vi "Local qubit state.vi"(11 "Circuit cluster":T1) -> (3 "Local qubit state":cdb[](array[numeric]))   [LabVIEW 2016]
doc: "*Local state vector is only valid for non-entangled qubits"
uses:
  TypeDefs/Circuit Cluster.ctl
  Classes/GateAbst/GateAbst.lvclass
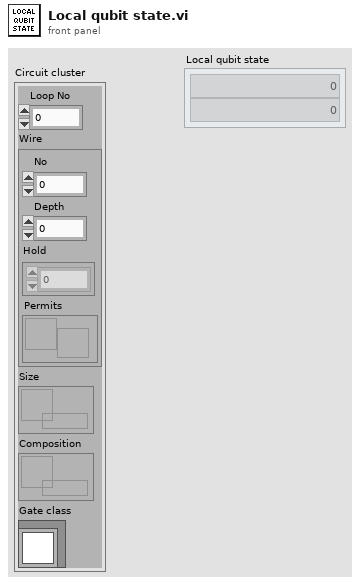
[diagram p1: front panel]
types:
  T1 = typedef "Circuit Cluster.ctl" = cluster{"Loop No":i32, "Wire":cluster{"No":i32, "Depth":i32, "Hold":i32[][], "Permits":refnum<notifier>}, "Size":refnum<queue>, "Composition":refnum<queue>, "Gate class":refnum<class "GateAbst.lvclass">}
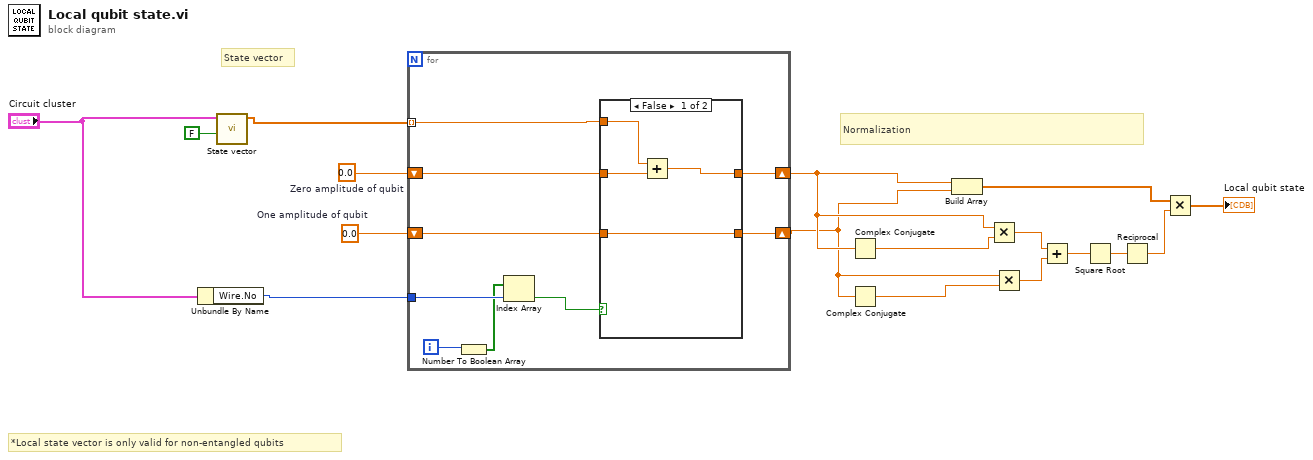
[diagram p0: block diagram]
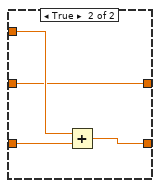
[diagram p2: hidden frame]
diagram:
  w14 = 0.0  # One amplitude of qubit
  w15 = 0.0  # Zero amplitude of qubit
  # "*Local state vector is only valid for non-entangled qubits"
  # "Normalization"
  # "State vector"
  n1 = Unbundle By Name("Circuit cluster") -> ("Wire.No"=w17:i32)
  n2 = call "State vector.vi"("Final state? (T)"=FALSE ("Final state?"), "Circuit cluster"="Circuit cluster") -> ("State vector"=w3:cdb[])  [unwired: 9 in]
  n3 = for {
    tunnel: w17 -> [w25]
    tunnel: w3 -> [w22] mode=indexing
    shift-right: [w18] -> w10
    shift-left: w14 -> [w19]
    shift-right: [w20] -> w11
    shift-left: w15 -> [w21]
    i -> [w26]
    n4 = Number To Boolean Array(number=w26) -> (Boolean array=w24:bool[])
    n5 = Index Array "Index Array"(array=w24, index=w25) -> (element=w23:bool)
    n6 = case shown="False" w23 {
      tunnel: w22 -> [w30 w34]
      tunnel: w21 -> [w29 w31]
      tunnel: [w28 w31] -> w20
      tunnel: w19 -> [w27 w33]
      tunnel: [w27 w32] -> w18
      frame False {
        n7 = Add(x=w30, y=w29) -> (x+y=w28:cdb)
      }
      frame True {
        n8 = Add(x=w34, y=w33) -> (x+y=w32:cdb)
      }
    }
  }
  n9 = Complex Conjugate(1:w11) -> (0:w16:cdb)
  n10 = Complex Conjugate(1:w10) -> (0:w13:cdb)
  n11 = Build Array "Build Array"(w11, w10) -> (w7:cdb[])
  n12 = Multiply(x=w11, y=w16) -> (x*y=w5:cdb)
  n13 = Multiply(x=w10, y=w13) -> (x*y=w4:cdb)
  n14 = Add(x=w5, y=w4) -> (x+y=w12:cdb)
  n15 = Square Root(x=w12) -> (sqrt(x)=w8:cdb)
  n16 = Reciprocal(x=w8) -> (1/x=w9:cdb)
  n17 = Multiply(x=w7, y=w9) -> (x*y=→"Local qubit state":cdb[])
